vi "getAdditionalDataXML.vi"(8 "error in (no error)":errorcluster, 11 "SingleTone in":refnum<class "SingleTone.lvclass">) -> (0 "error out":errorcluster, 2 "additionalDataXML":refnum<class "xmlNode.lvclass">, 3 "SingleTone out":refnum<class "SingleTone.lvclass">)   [LabVIEW 2009, in "Tools.lvlib" / "Scripting.lvlib" / "SingleTone.lvclass"]
uses:
  SingleTone.lvclass
  xmlNode/xmlNode.lvclass
  SingleTone.lvclass/SingleTone.ctl
  ScriptEvent.lvclass
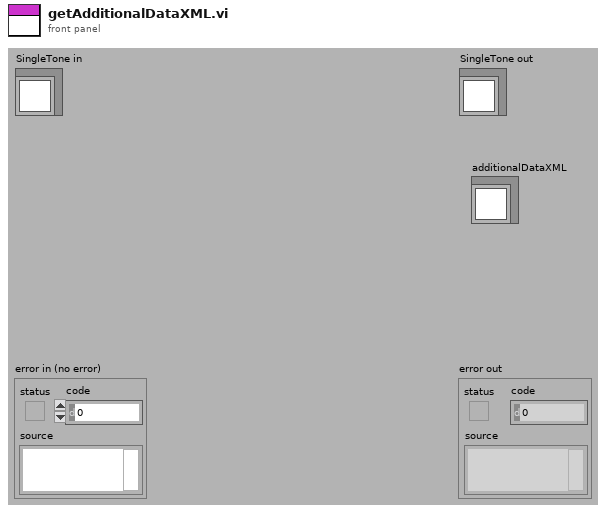
[diagram p1: front panel]
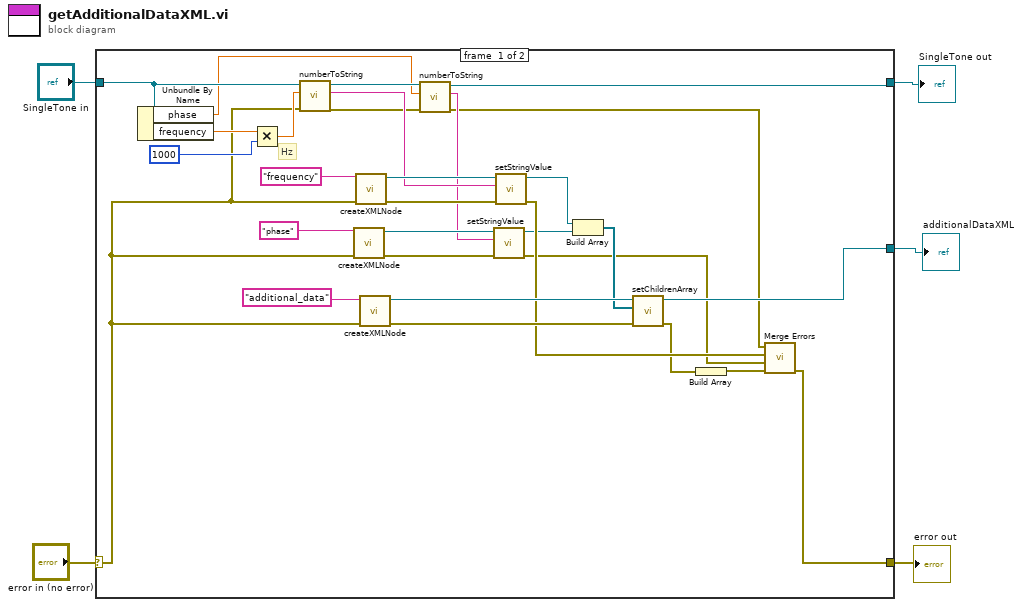
[diagram p0: block diagram]
diagram:
  n1 = case shown="No Error" "error in (no error)" {
    selector: "error in (no error)" -> [w16 w36]
    tunnel: [w23 w36] -> w4
    tunnel: [w6 w37] -> w3
    tunnel: "SingleTone in" -> [w32 w37]
    tunnel: [w25 _] -> w1
    frame #0 {
      # "Hz"
      n2 = Unbundle By Name(w32) -> ("phase"=w13:dbl, "frequency"=w22:dbl)
      n3 = Multiply(x=w22, y=1000) -> (x*y=w21:dbl)
      n4 = call "numberToString.vi"("error in (no error)"=w16, "Numeric"=w21, "ScriptEvent in"=w32) -> ("error out"=w15:errorcluster, "String"=w31:string, "ScriptEvent out"=w14:refnum<class "SingleTone.lvclass">)  [unwired: 6 in]
      n5 = call "createXMLNode.vi"("error in (no error)"=w16, "name"="phase") -> ("error out"=w17:errorcluster, "xmlNode out"=w18:refnum<class "xmlNode.lvclass">)  [unwired: 8 in]
      n6 = call "createXMLNode.vi"("error in (no error)"=w16, "name"="frequency") -> ("error out"=w33:errorcluster, "xmlNode out"=w34:refnum<class "xmlNode.lvclass">)  [unwired: 8 in]
      n7 = call "createXMLNode.vi"("error in (no error)"=w16, "name"="additional_data") -> ("error out"=w28:errorcluster, "xmlNode out"=w30:refnum<class "xmlNode.lvclass">)  [unwired: 8 in]
      n8 = call "numberToString.vi"("error in (no error)"=w15, "Numeric"=w13, "ScriptEvent in"=w14) -> ("error out"=w9:errorcluster, "String"=w12:string, "ScriptEvent out"=w6:refnum<class "SingleTone.lvclass">)  [unwired: 6 in]
      n9 = call-dynamic "setStringValue.vi"("error in (no error)"=w17, "stringValue"=w12, "xmlNode.lvclass in"=w18) -> ("error out"=w10:errorcluster, "xmlNode.lvclass out"=w11:refnum<class "xmlNode.lvclass">)  [unwired: 7 in]
      n10 = call-dynamic "setStringValue.vi"("error in (no error)"=w33, "stringValue"=w31, "xmlNode.lvclass in"=w34) -> ("error out"=w24:errorcluster, "xmlNode.lvclass out"=w27:refnum<class "xmlNode.lvclass">)  [unwired: 7 in]
      n11 = Build Array(w27, w11) -> (w26:refnum<class "xmlNode.lvclass">[])
      n12 = call-dynamic "setChildrenArray.vi"("error in (no error)"=w28, "Children"=w26, "xmlNode.lvclass in"=w30) -> ("error out"=w7:errorcluster, "xmlNode.lvclass out"=w25:refnum<class "xmlNode.lvclass">)  [unwired: 7 in]
      n13 = Build Array(w7) -> (w8:errorcluster[])
      n14 = call <vilib>:"Merge Errors.vi"("error array in"=w8, "error in 3 (no error)"=w10, "error in 2 (no error)"=w24, "error in 1 (no error)"=w9) -> ("error out"=w23:errorcluster)  [unwired: 3 in]
    }
    frame #1 {
    }
  }
  "error out" <- w4
  "SingleTone out" <- w3
  "additionalDataXML" <- w1
